vi "Teleop.vi"(10 "Match Info":T2={"Autonomous Elapsed Seconds"=0.0, "TeleOp Elapsed Seconds"=0.0, "Disabled Elapsed Seconds"=0.0, "Visited Autonomous"=FALSE, "Visited TeleOp"=FALSE, "Visited Disabled"=FALSE, "Autonomous Settings"={"Autonomous Style"=enum."Independent", "VI Refnum"=refnum}}, 11 "Call Context":T3) -> ()   [LabVIEW 2016]
doc: "This VI is called for each TeleOp packet received from the DS where the robot is not disabled. It is often used to read from the joysticks and update I/O or to update setpoints for timed control loops. It should complete and return within 20 milliseconds or it may miss DS packets."
uses:
  <vilib>/Rock Robotics/WPI/DriverStation/WPI_DriverStationDerivedRobotMode.ctl
  <vilib>/Rock Robotics/WPI/DriverStation/WPI_DriverStationMatch Info.ctl
  Robot Global Data.vi
  <vilib>/Rock Robotics/WPI/Utilities/WPI_GetSetVariantRefNum.vi
  <vilib>/Rock Robotics/WPI/Solenoid/Deprecated/WPI_SolenoidSetBool.vi
  <vilib>/addons/control/pid/pid.llb/PID (DBL).vi
  navX Library v2/navX Library v2.lvlib
  <vilib>/addons/control/pid/NI_PID_pid.lvlib
panel:
  in  "MOE":dbl=25.0 format="%#_13g"
  in  "Center":dbl=180.0 format="%#_13g"
  out "out left":dbl
  out "out right":dbl
  in  "Pid Factor":dbl=8400.0
  in  "Mode":bool=TRUE
  in  "output range":cluster{"output high":dbl, "output low":dbl}={"output high"=1.0, "output low"=-1.0} {"output low" format="%.2f"; "output high" format="%.2f"}
  in  "PID gains":T1={"proportional gain (Kc)"=0.00021, "integral time (Ti, min)"=15.0, "derivative time (Td, min)"=0.0} {"derivative time (Td, min)" format="%.6f"; "integral time (Ti, min)" format="%.6f"; "proportional gain (Kc)" format="%.6f"}
  out "Left":dbl(graph)
  out "Right":dbl(graph)
  out "Encoder Right":dbl(graph)
  out "Encoder Left":dbl(graph)
  in  "Speed":dbl=0.45 format="%#_13g"
  out "Out Left":dbl(graph)
  out "Out Right":dbl(graph)
  out "Shooter":cluster{"Sensor Velocity":dbl, dbl, dbl}(graph)
  in  "ShooterRPM":dbl
  in  "P":dbl=0.5 format="%#_13g"
  in  "I":dbl format="%#_13g"
  in  "D":dbl format="%#_13g"
  in  "F":dbl=0.005212 format="%#_13g"
  in  "I Zone":dbl format="%#_13g"
  in  "Ramp Rate":dbl format="%#_13g"
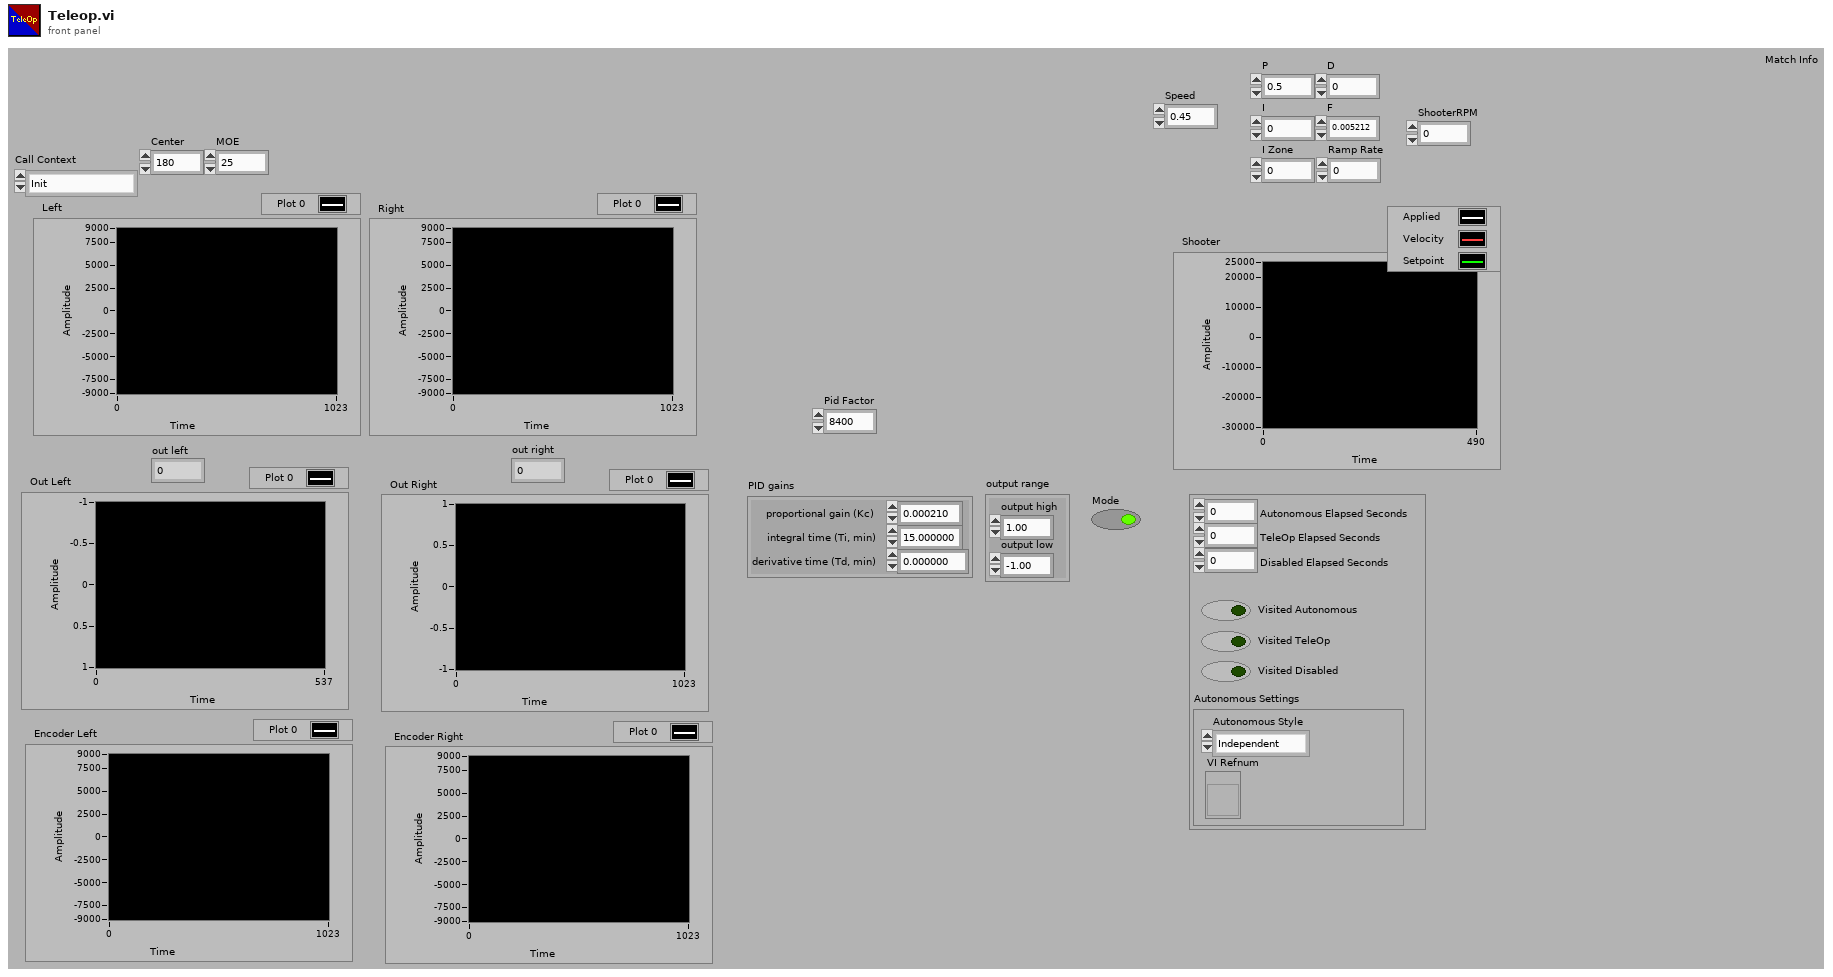
[diagram p1: front panel]
types:
  T1 = cluster{"proportional gain (Kc)":dbl, "integral time (Ti, min)":dbl, "derivative time (Td, min)":dbl}
  T2 = typedef "WPI_DriverStationMatch Info.ctl" = cluster{"Autonomous Elapsed Seconds":dbl, "TeleOp Elapsed Seconds":dbl, "Disabled Elapsed Seconds":dbl, "Visited Autonomous":bool, "Visited TeleOp":bool, "Visited Disabled":bool, "Autonomous Settings":cluster{"Autonomous Style":enum16{"Iterative", "Independent"}, "VI Refnum":refnum<vi>}}
  T3 = typedef "WPI_DriverStationDerivedRobotMode.ctl" = enum16{"Init", "Execute", "Stop"}
  T4 = typedef "WPI_SolenoidDevRef.ctl" = cluster{"DevStatus":errorcluster, "Pneumatics Control Module":u8, "Forward Solenoid Channel":T5, "Reverse Solenoid Channel":T5}
  T5 = typedef "WPI_SolenoidChannel.ctl" = enum8{"Solenoid 0", "Solenoid 1", "Solenoid 2", "Solenoid 3", "Solenoid 4", "Solenoid 5", "Solenoid 6", "Solenoid 7", "Invalid"}
  T6 = typedef "WPI_JoystickDevRef.ctl" = cluster{"Device":T7}
  T7 = typedef "WPI_JoystickDeviceEnum.ctl" = enum16{"USB 0", "USB 1", "USB 2", "USB 3", "USB 4", "USB 5"}
  T8 = cluster{"Buttons[0]":bool, "Buttons[1]":bool, "Buttons[2]":bool, "Buttons[3]":bool, "Buttons[4]":bool, "Buttons[5]":bool, "Buttons[6]":bool, "Buttons[7]":bool, "Buttons[8]":bool}
  T9 = cluster{"Axes[0]":dbl, "Axes[1]":dbl, "Axes[2]":dbl, "Axes[3]":dbl, "Axes[4]":dbl, "Axes[5]":dbl, "Axes[6]":dbl, "Axes[7]":dbl, "Axes[8]":dbl}
  T10 = typedef "navX Library v2.lvlib/Z900_navX_DeviceTypeDef.ctl" = cluster{"Interface":cluster{"Protocol":T11, "Update Rate (4Hz-100Hz)":u8, "navX Open TypeDef":variant}, "Notify Packet":refnum<notifier>, "Loop VI Refnum":refnum<vi>, "Ready to Close Occurrence Refnum":refnum<k4>}
  T11 = typedef "navX Library v2.lvlib/Z900_navX_ProtocolTypeDef.ctl" = enum16{"SERIAL", "I2C", "SPI"}
  T12 = cluster{"Velocity X":dbl, "Velocity Y":dbl, "Velocity Z":dbl, "Displacement X":dbl, "Displacement Y":dbl, "Displacement Z":dbl}
  T13 = cluster{"LinearAcceleration X":dbl, "LinearAcceleration Y":dbl, "LinearAcceleration Z":dbl}
  T14 = cluster{"Yaw":dbl, "Roll":dbl, "Pitch":dbl, "Heading":dbl, "Fused Heading":dbl}
  T15 = typedef "WPI_MotorControlDeviceRef.ctl" = cluster{"DeviceStatus":errorcluster, "Type":T16, "PWM":cluster{"PWM Channel":T17, "DeadBand":T18}, "CAN":cluster{"Device Number":u8, "SetOutput VI Ref":variant, "GetOutput VI Ref":variant, "Enable VI Ref":variant, "Disable VI Ref":variant, "Data":variant}, "Invert":bool}
  T16 = typedef "WPI_MotorControlType.ctl" = enum16{"PWM", "CAN"}
  T17 = typedef "FPGA_DIOPWMChannel.ctl" = enum8{"PWM 0", "PWM 1", "PWM 2", "PWM 3", "PWM 4", "PWM 5", "PWM 6", "PWM 7", "PWM 8", "PWM 9", "PWM MXP 0", "PWM MXP 1", "PWM MXP 2", "PWM MXP 3", "PWM MXP 4", "PWM MXP 5", "PWM MXP 6", "PWM MXP 7", "PWM MXP 8", "PWM MXP 9", "Invalid"}
  T18 = typedef "WPI_PWMDeadband.ctl" = cluster{"Name":string, "maxPositivePwm":i32, "minPositivePwm":i32, "centerPwm":i32, "maxNegativePwm":i32, "minNegativePwm":i32, "angularRange":u16}
  T19 = typedef "WPI_CANTalonSRX_GlobalStatus.ctl" = cluster{"Applied Throttle":dbl, "Module Enabled":bool, "CAN Error":errorcluster, "Closed Loop Error":dbl, "Forward Limit Switch Closed":bool, "Reverse Limit Switch Closed":bool, "Sensor Position":dbl, "Sensor Velocity":dbl, "Current":dbl, "Sticky Fault - Over Temp":bool, "Sticky Fault - Under Voltage":bool, "Sticky Fault - Forward Limit":bool, "Sticky Fault - Reverse Limit":bool, "Sticky Fault - Forward Soft Limit":bool, "Sticky Fault - Reverse Soft Limit":bool, "Brake is Enabled":bool, "Encoder Position":dbl, "Encoder Velocity":dbl, "Encoder Index Count":dbl, "Encoder A Pin State":bool, "Encoder B Pin State":bool, "Encoder Index Pin State":bool, "Analog In":dbl, "Analog In Velocity":dbl, "Temperature (C)":dbl, "Battery Voltage":dbl, "Control 5 Is Supported":bool, "Current Profile Slot Select":dbl, "Pos Div 8":bool, "Vel Div 4":bool, "Pulse Width Position":i32, "Pulse Width Velocity":i32, "Pulse Width Rise To Rise (us)":i32, "Pulse Width Rise To Fall (us)":i32, "Mot Prof Active Is Under Run":bool, "Mot Prof Active Has Under Run":bool, "Mot Prof Active Is Last":bool, "Mot Prof Active Velocity Only":bool, "Mot Prof Active Is Valid":bool, "Mot Prof Buffer Is Full":bool, "Mot Prof Active Profile Slot Select":i32, "Mot Prof NextID":i32, "Mot Prof Count":i32, "Mot Prof Active Velocity":dbl, "Mot Prof Active Position":dbl, "Mot Prof Output Enable":i32}
  T20 = cluster{dbl, "Sensor Velocity":dbl, "ShooterRPM":dbl}
  T21 = typedef "WPI_EncoderDevRef.ctl" = cluster{"DevStatus":errorcluster, "EncoderIndex":T22, "CounterIndex":T23, "DistancePerCount":dbl, "Decoding Type":T24}
  T22 = typedef "FPGA_EncoderIdx.ctl" = enum8{"Enc 0", "Enc 1", "Enc 2", "Enc 3", "Enc 4", "Enc 5", "Enc 6", "Enc 7", "Invalid"}
  T23 = typedef "FPGA_CounterCtrSystemIndex.ctl" = enum8{"Ctr 0", "Ctr 1", "Ctr 2", "Ctr 3", "Ctr 4", "Ctr 5", "Ctr 6", "Ctr 7", "Invalid"}
  T24 = typedef "WPI_EncoderType.ctl" = enum16{"1x", "2x", "4x"}
  T25 = typedef "WPI_RobotDriveDevRef.ctl" = cluster{"DevStatus":errorcluster, "Motors[]":T15[], "Square Inputs":bool, "Max Output":dbl}
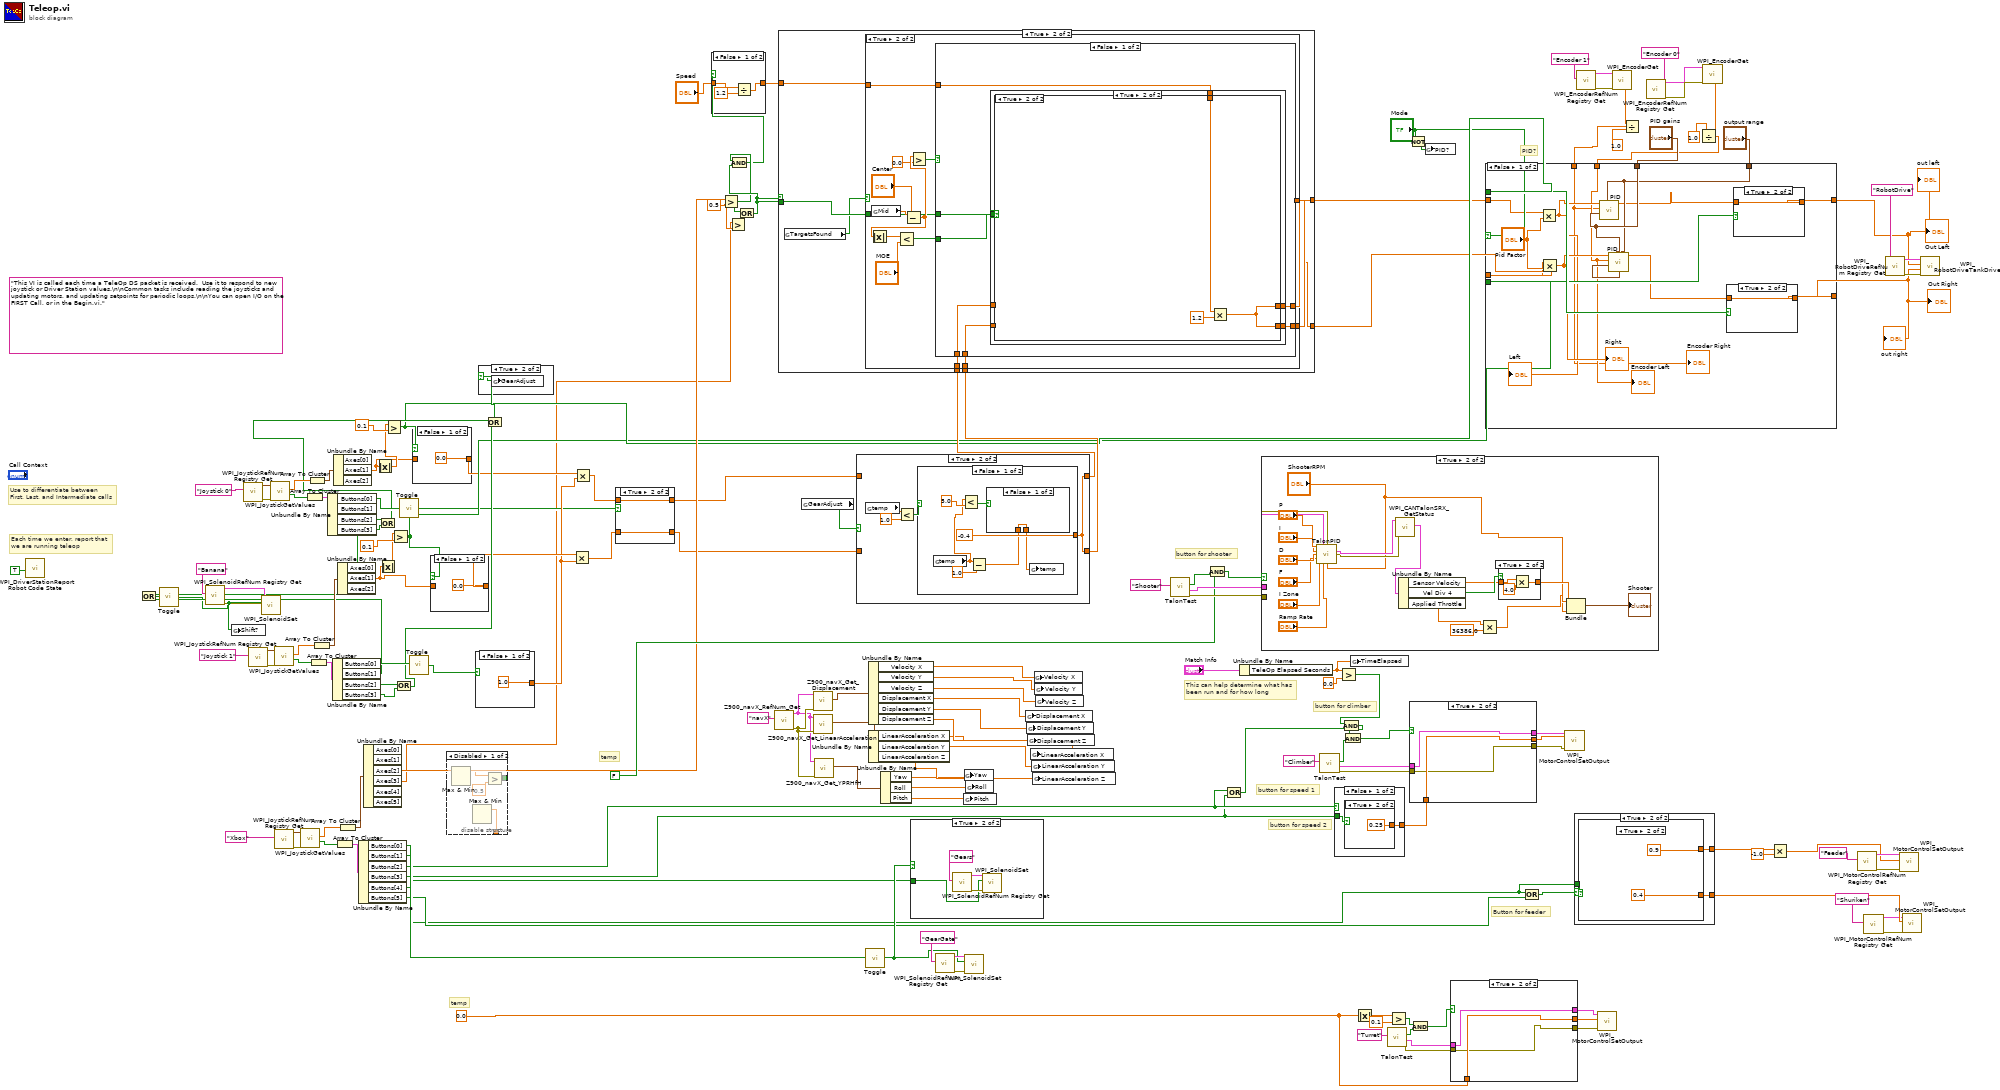
[diagram p0: block diagram]
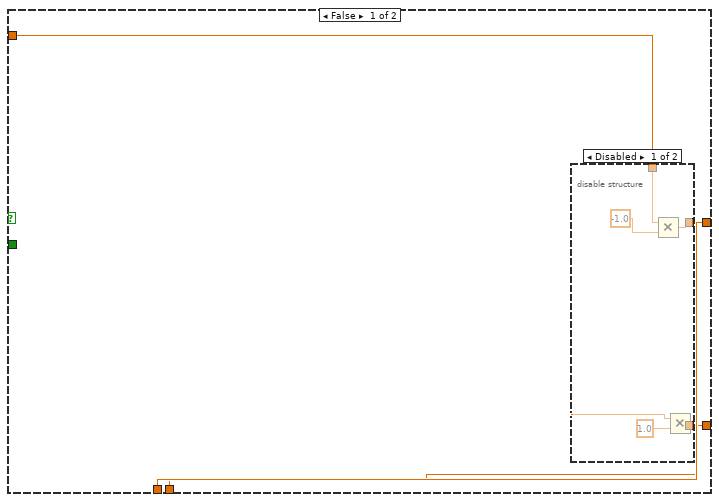
[diagram p4: hidden frame]
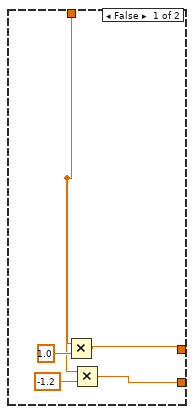
[diagram p7: hidden frame]
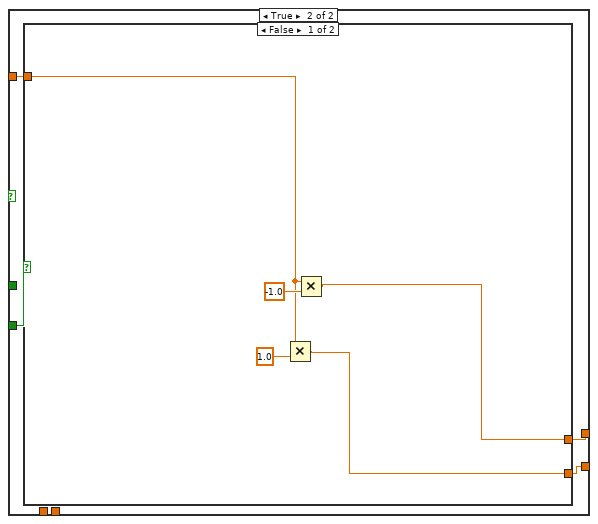
[diagram p8: hidden frame]
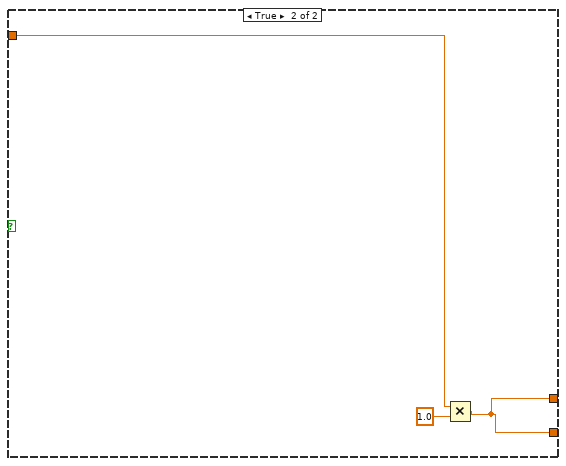
[diagram p9: hidden frame]
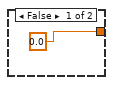
[diagram p10: hidden frame]
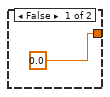
[diagram p11: hidden frame]
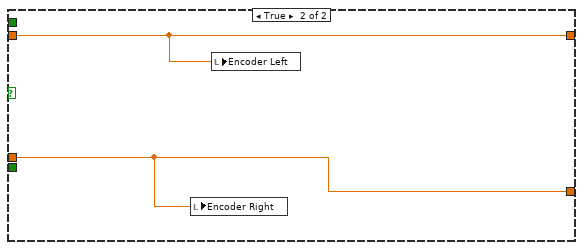
[diagram p12: hidden frame]
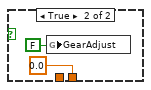
[diagram p16: hidden frame]
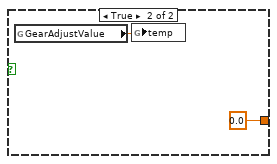
[diagram p17: hidden frame]
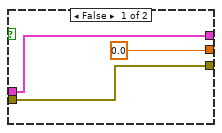
[diagram p18: hidden frame]
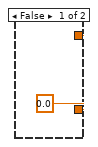
[diagram p20: hidden frame]
diagram:
  w12 = 0.5 ("y")
  w66 = 0.0
  (unwired) "This VI is called each time a TeleOp DS packet is received.  Use it to respond to new joystick or Driver Station values.\n\nCommon tasks include reading the joysticks and updating motors, and updating setpoints for periodic loops.\n\nYou can open I/O on the FIRST Call, or in the Begin.vi."
  # "PID?"
  # "temp"
  # "temp"
  # "Button for feeder"
  # "button for speed 2"
  # "button for speed 1"
  # "button for climber"
  # "button for shooter"
  # "Each time we enter, report that\nwe are running teleop"
  # "Use to differentiate between\nFirst, Last, and Intermediate calls"
  # "This can help determine what has\nbeen run and for how long"
  n1 = call <vilib>:"WPI_DriverStationReport Robot Code State.vi"("TeleOp"=TRUE ("Autonomous")) -> ()  [unwired: 10 in, 1 out]
  n2 = call <vilib>:"WPI_SolenoidRefNum Registry Get.vi"("refnum name"="Banana") -> ("error out"=w20:errorcluster, "SolenoidDevRef"=w19:T4)  [unwired: 9 in]
  n3 = call <vilib>:"WPI_JoystickRefNum Registry Get.vi"("refnum name"="Joystick 0") -> ("error out"=w161:errorcluster, "JoystickDevRef"=w160:T6)  [unwired: 9 in]
  n4 = call <vilib>:"WPI_JoystickRefNum Registry Get.vi"("refnum name"="Joystick 1") -> ("error out"=w153:errorcluster, "JoystickDevRef"=w152:T6)  [unwired: 9 in]
  n5 = call <vilib>:"WPI_JoystickGetValues.vi"("error in (no error)"=w161, "JoystickDevRef"=w160) -> ("Buttons"=w157:bool[], "Axes"=w158:dbl[])  [unwired: 5 in, 3 out]
  n6 = call <vilib>:"WPI_JoystickRefNum Registry Get.vi"("refnum name"="Xbox") -> ("error out"=w113:errorcluster, "JoystickDevRef"=w112:T6)  [unwired: 9 in]
  n7 = call <vilib>:"WPI_JoystickGetValues.vi"("error in (no error)"=w153, "JoystickDevRef"=w152) -> ("Buttons"=w149:bool[], "Axes"=w150:dbl[])  [unwired: 5 in, 3 out]
  n8 = call <vilib>:"WPI_JoystickGetValues.vi"("error in (no error)"=w113, "JoystickDevRef"=w112) -> ("Buttons"=w109:bool[], "Axes"=w110:dbl[])  [unwired: 5 in, 3 out]
  n9 = Array To Cluster(array=w157) -> (cluster=w155:T8)
  n10 = Array To Cluster(array=w158) -> (cluster=w156:T9)
  n11 = Array To Cluster(array=w149) -> (cluster=w147:T8)
  n12 = Array To Cluster(array=w150) -> (cluster=w148:T9)
  n13 = Unbundle By Name(w155) -> ("Buttons[0]"=w141:bool, "Buttons[1]"=w15:bool, "Buttons[2]"=w72:bool, "Buttons[3]"=w71:bool)
  n14 = Unbundle By Name(w147) -> ("Buttons[0]"=w140:bool, "Buttons[1]"=w16:bool, "Buttons[2]"=w74:bool, "Buttons[3]"=w73:bool)
  n15 = Or(x=w15, y=w16) -> (x .or. y?=w17:bool)
  n16 = call "Toggle.vi"("Input"=w17) -> ("Output"=w2:bool)
  n17 = global write "Robot Global Data.vi" "Shift?"(w2) -> ()
  n18 = call-poly <vilib>:"WPI_SolenoidSet.vi"("error in (no error)"=w20, "Value"=w2, "SolenoidDevRef"=w19) -> ()  [unwired: 7 in, 2 out]
  n19 = Unbundle By Name(w156) -> ("Axes[1]"=w142:dbl)  [unwired: 2 out]
  n20 = Array To Cluster(array=w109) -> (cluster=w107:T8)
  n21 = Unbundle By Name(w148) -> ("Axes[1]"=w144:dbl)  [unwired: 2 out]
  n22 = Array To Cluster(array=w110) -> (cluster=w108:T9)
  n23 = Unbundle By Name(w107) -> ("Buttons[0]"=w106:bool, "Buttons[1]"=w105:bool, "Buttons[2]"=w104:bool, "Buttons[3]"=w103:bool, "Buttons[4]"=w100:bool, "Buttons[5]"=w101:bool)
  n24 = Unbundle By Name(w108) -> ("Axes[2]"=w64:dbl, "Axes[3]"=w11:dbl)  [unwired: 4 out]
  n25 = Absolute Value(x=w142) -> (abs(x)=w143:dbl)
  n26 = Or(x=w72, y=w71) -> (x .or. y?=w70:bool)
  n27 = Absolute Value(x=w144) -> (abs(x)=w145:dbl)
  n28 = Greater?(x=w143, y=0.1 ("x")) -> (0:w55:bool)
  n29 = Greater?(x=w145, y=0.1 ("x")) -> (0:w54:bool)
  n30 = Or(x=w74, y=w73) -> (x .or. y?=w69:bool)
  n31 = call "Toggle.vi"("Input"=w141) -> ("Output"=w46:bool)
  n32 = call "Toggle.vi"("Input"=w140) -> ("Output"=w139:bool)
  n33 = case shown="False" w55 {
    tunnel: w142 -> [_ w164]
    tunnel: [0.0 w164] -> w51
    frame False {
    }
    frame True {
    }
  }
  n34 = case shown="False" w54 {
    tunnel: w144 -> [_ w166]
    tunnel: [0.0 w166] -> w53
    frame False {
    }
    frame True {
    }
  }
  n35 = disable-structure shown="Disabled" {
    disable-tunnel: [w168 _] -> _
    disable-tunnel: [w167 _] -> _
    frame Disabled {
      n36 = Max & Min() -> (max(x,y)=w170:dbl)  [unwired: 2 in, 1 out]
      n37 = Max & Min() -> (max(x,y)=w167:dbl)  [unwired: 2 in, 1 out]
      n38 = Greater?(x=w170, y=0.5) -> (0:w168:bool)
    }
    frame Enabled {
    }
  }
  n39 = case shown="False" w139 {
    tunnel: [1.0 0.8] -> w52
    frame False {
    }
    frame True {
    }
  }
  n40 = Or(x=w70, y=w69) -> (x .or. y?=w67:bool)
  n41 = case shown="True" w67 {
    selector: w67 -> [_ w173]
    frame False {
    }
    frame True {
      n42 = global write "Robot Global Data.vi" "GearAdjust"(w173) -> ()
    }
  }
  n43 = Multiply(x=w53, y=w52) -> (x*y=w49:dbl)
  n44 = Multiply(x=w51, y=w52) -> (x*y=w50:dbl)
  n45 = case shown="True" w46 {
    tunnel: w50 -> [w175 w180]
    tunnel: w49 -> [w174 w179]
    tunnel: [w178 w180] -> w48
    tunnel: [w177 w179] -> w47
    frame False {
      w176 = -1.0
      n46 = Multiply(x=w176, y=w175) -> (x*y=w177:dbl)
      n47 = Multiply(x=w174, y=w176) -> (x*y=w178:dbl)
    }
    frame True {
    }
  }
  n48 = Greater?(x=w64, y=w12) -> (0:w6:bool)
  n49 = Greater?(x=w11, y=w12) -> (0:w8:bool)
  n50 = Or(x=w6, y=w8) -> (x .or. y?=w7:bool)
  n51 = And(x=w6, y=w7) -> (x .and. y?=w5:bool)
  n52 = case shown="False" w5 {
    tunnel: [w183 w184] -> w10
    tunnel: "Speed" -> [w182 w184]
    frame False {
      n53 = Divide(x=w182, y=1.2) -> (x/y=w183:dbl)
    }
    frame True {
    }
  }
  n54 = call "Z900_navX_RefNum_Get.vi"("refnum name"="navX") -> ("error out"=w137:errorcluster, "navX Device"=w136:T10)  [unwired: 9 in]
  n55 = global read "Robot Global Data.vi" "GearAdjust"() -> (w68:bool)
  n56 = call "Z900_navX_Get_Displacement.vi"("error in (no error)"=w137, "navX Device"=w136) -> ("Displacement"=w133:T12)  [unwired: 6 in, 3 out]
  n57 = call "Z900_navX_Get_LinearAcceleration.vi"("error in (no error)"=w137, "navX Device"=w136) -> ("Linear Acceleration"=w134:T13)  [unwired: 6 in, 3 out]
  n58 = call "Z900_navX_Get_YPRHfH.vi"("error in (no error)"=w137, "navX Device"=w136) -> ("YRPHfH"=w135:T14)  [unwired: 6 in, 3 out]
  n59 = case shown="True" w68 {
    tunnel: w48 -> [w186 _]
    tunnel: w47 -> [w185 _]
    tunnel: [w186 w187] -> w60
    tunnel: [w185 w187] -> w59
    frame False {
    }
    frame True {
      n60 = global read "Robot Global Data.vi" "temp"() -> (w190:dbl)
      n61 = Less?(x=w190, y=1.0) -> (x < y?=w188:bool)
      n62 = case shown="False" w188 {
        tunnel: [-0.4 0.0] -> w187
        frame False {
          n63 = global read "Robot Global Data.vi" "temp"() -> (w193:dbl)
          n64 = Less?(x=w193, y=5.0 ("x")) -> (x < y?=w194:bool)
          n65 = Subtract(x=w193, y=1.0) -> (x-y=w191:dbl)
          n66 = case shown="False" w194 {
            tunnel: [w198 0.0] -> w192
            tunnel: w191 -> [w198 _]
            frame False {
            }
            frame True {
              n67 = global write "Robot Global Data.vi" "GearAdjust"(FALSE) -> ()
            }
          }
          n68 = global write "Robot Global Data.vi" "temp"(w192) -> ()
        }
        frame True {
          n69 = global read "Robot Global Data.vi" "GearAdjustValue"() -> (w202:dbl)
          n70 = global write "Robot Global Data.vi" "temp"(w202) -> ()
        }
      }
    }
  }
  n71 = case shown="True" w7 {
    tunnel: w60 -> [w204 w211]
    tunnel: w59 -> [w203 w210]
    tunnel: w7 -> [_ w209]
    tunnel: [w204 w207] -> w13
    tunnel: [w203 w206] -> w14
    tunnel: w10 -> [_ w205]
    frame False {
    }
    frame True {
      n72 = global read "Robot Global Data.vi" "TargetsFound"() -> (w208:bool)
      n73 = case shown="True" w208 {
        tunnel: w211 -> [w213 w228]
        tunnel: w210 -> [w212 w227]
        tunnel: [w212 w226] -> w207
        tunnel: [w213 w225] -> w206
        tunnel: w209 -> [_ w221]
        tunnel: w205 -> [w214 w220]
        frame False {
          n74 = disable-structure shown="Disabled" {
            disable-tunnel: [w218 _] -> _
            disable-tunnel: [w217 _] -> _
            disable-tunnel: w214 -> [w215 _]
            frame Disabled {
              n75 = Multiply(x=w215, y=-1.0) -> (x*y=w218:dbl)
              n76 = Multiply(x=w215, y=1.0) -> (x*y=w217:dbl)
            }
            frame Enabled {
            }
          }
        }
        frame True {
          n77 = global read "Robot Global Data.vi" "Mid"() -> (w233:dbl)
          n78 = Subtract(x=w233, y="Center") -> (x-y=w223:dbl)
          n79 = Absolute Value(x=w223) -> (abs(x)=w231:dbl)
          n80 = Less?(x=w231, y="MOE") -> (x < y?=w229:bool)
          n81 = Greater?(x=w223, y=0.0) -> (0:w224:bool)
          n82 = case shown="False" w224 {
            tunnel: w229 -> [w240 w258]
            tunnel: w228 -> [w239 _]
            tunnel: w227 -> [w238 _]
            tunnel: [w237 w256] -> w226
            tunnel: [w236 w257] -> w225
            tunnel: w221 -> [w235 _]
            tunnel: w220 -> [w234 w255]
            frame False {
              n83 = case shown="True" w235 {
                tunnel: w240 -> [_ w246]
                tunnel: w239 -> [w242 _]
                tunnel: w238 -> [w241 _]
                tunnel: [w242 w245] -> w236
                tunnel: [w241 w244] -> w237
                tunnel: w234 -> [_ w243]
                frame False {
                }
                frame True {
                  n84 = case shown="True" w246 {
                    tunnel: [w251 w254] -> w245
                    tunnel: [w249 w254] -> w244
                    tunnel: w243 -> [w247 w252]
                    frame False {
                      n85 = Multiply(x=w247, y=1.0) -> (x*y=w251:dbl)
                      n86 = Multiply(x=w247, y=-1.2) -> (x*y=w249:dbl)
                    }
                    frame True {
                      n87 = Multiply(x=w252, y=1.2) -> (x*y=w254:dbl)
                    }
                  }
                }
              }
            }
            frame True {
              n88 = case shown="False" w258 {
                tunnel: [w263 w266] -> w257
                tunnel: [w261 w266] -> w256
                tunnel: w255 -> [w259 w264]
                frame False {
                  n89 = Multiply(x=w259, y=1.0) -> (x*y=w261:dbl)
                  n90 = Multiply(x=w259, y=-1.0) -> (x*y=w263:dbl)
                }
                frame True {
                  n91 = Multiply(x=w264, y=1.0) -> (x*y=w266:dbl)
                }
              }
            }
          }
        }
      }
    }
  }
  n92 = call "Toggle.vi"("Input"=w106) -> ("Output"=w114:bool)
  n93 = Unbundle By Name(w133) -> ("Velocity X"=w45:dbl, "Velocity Y"=w44:dbl, "Velocity Z"=w43:dbl, "Displacement X"=w42:dbl, "Displacement Y"=w41:dbl, "Displacement Z"=w40:dbl)
  n94 = Unbundle By Name(w134) -> ("LinearAcceleration X"=w39:dbl, "LinearAcceleration Y"=w38:dbl, "LinearAcceleration Z"=w37:dbl)
  n95 = Unbundle By Name(w135) -> ("Yaw"=w36:dbl, "Roll"=w35:dbl, "Pitch"=w34:dbl)
  n96 = case shown="True" w114 {
    tunnel: w105 -> [_ w267]
    frame False {
    }
    frame True {
      n97 = call <vilib>:"WPI_SolenoidRefNum Registry Get.vi"("refnum name"="Gears") -> ("error out"=w270:errorcluster, "SolenoidDevRef"=w269:T4)  [unwired: 9 in]
      n98 = call-poly <vilib>:"WPI_SolenoidSet.vi"("error in (no error)"=w270, "Value"=w267, "SolenoidDevRef"=w269) -> ()  [unwired: 7 in, 2 out]
    }
  }
  n99 = call <vilib>:"WPI_SolenoidRefNum Registry Get.vi"("refnum name"="GearGate") -> ("error out"=w117:errorcluster, "SolenoidDevRef"=w116:T4)  [unwired: 9 in]
  n100 = global write "Robot Global Data.vi" "Pitch"(w34) -> ()
  n101 = global write "Robot Global Data.vi" "Yaw"(w36) -> ()
  n102 = call-poly <vilib>:"WPI_SolenoidSet.vi"("error in (no error)"=w117, "Value"=w114, "SolenoidDevRef"=w116) -> ()  [unwired: 7 in, 2 out]
  n103 = global write "Robot Global Data.vi" "Roll"(w35) -> ()
  n104 = global write "Robot Global Data.vi" "Displacement X"(w42) -> ()
  n105 = global write "Robot Global Data.vi" "Displacement Y"(w41) -> ()
  n106 = global write "Robot Global Data.vi" "Displacement Z"(w40) -> ()
  n107 = global write "Robot Global Data.vi" "LinearAcceleration X"(w39) -> ()
  n108 = global write "Robot Global Data.vi" "LinearAcceleration Y"(w38) -> ()
  n109 = global write "Robot Global Data.vi" "LinearAcceleration Z"(w37) -> ()
  n110 = global write "Robot Global Data.vi" "Velocity X"(w45) -> ()
  n111 = global write "Robot Global Data.vi" "Velocity Y"(w44) -> ()
  n112 = global write "Robot Global Data.vi" "Velocity Z"(w43) -> ()
  n113 = call "TalonTest.vi"("Name"="Shooter") -> ("Output"=w127:bool, "Ref"=w131:T15, "error out"=w130:errorcluster)  [unwired: 7 in]
  n114 = And(x=FALSE, y=w127) -> (x .and. y?=w128:bool)
  n115 = Or(x=w104, y=w103) -> (x .or. y?=w102:bool)
  n116 = Unbundle By Name("Match Info") -> ("TeleOp Elapsed Seconds"=w4:dbl)
  n117 = case shown="True" w128 {
    tunnel: w131 -> [_ w275]
    tunnel: w130 -> [_ w271]
    frame False {
    }
    frame True {
      n118 = call "TalonPID.vi"("P"="P", "Ref In"=w275, "Error in"=w271, "I"="I", "D"="D", "F"="F", "I Zone"="I Zone", "Ramp Rate"="Ramp Rate", "Output"="ShooterRPM") -> ("Ref Out"=w274:T15, "error out"=w273:errorcluster)  [unwired: 5 in]
      n119 = call <vilib>:"WPI_CANTalonSRX_GetStatus.vi"("error in (no error)"=w273, "CAN Talon SRX Ref"=w274) -> ("Talon SRX Status"=w289:T19)  [unwired: 7 in, 2 out]
      n120 = Unbundle By Name(w289) -> ("Sensor Velocity"=w287:dbl, "Vel Div 4"=w288:bool, "Applied Throttle"=w284:dbl)
      n121 = Multiply(x=w284, y=36386.0) -> (x*y=w283:dbl)
      n122 = case shown="True" w288 {
        tunnel: w287 -> [w290 w292]
        tunnel: [w290 w293] -> w282
        frame False {
        }
        frame True {
          n123 = Multiply(x=w292, y=4.0) -> (x*y=w293:dbl)
        }
      }
      n124 = Bundle(w283, "Sensor Velocity"=w282, "ShooterRPM"="ShooterRPM") -> (→"Shooter":T20)  [unwired: 1 in]
    }
  }
  n125 = call "TalonTest.vi"("Name"="Climber") -> ("Output"=w125:bool, "Ref"=w120:T15, "error out"=w119:errorcluster)  [unwired: 7 in]
  n126 = case shown="False" w104 {
    tunnel: [w295 w299] -> w118
    tunnel: w103 -> [w294 w298]
    frame False {
      n127 = case shown="True" w294 {
        tunnel: [0.0 0.25] -> w295
        frame False {
        }
        frame True {
        }
      }
    }
    frame True {
      n128 = case shown="True" w298 {
        tunnel: [0.75 1.0] -> w299
        frame False {
        }
        frame True {
        }
      }
    }
  }
  n129 = Greater?(x=w4, y=0.0) -> (0:w122:bool)
  n130 = And(x=w122, y=w102) -> (x .and. y?=w126:bool)
  n131 = And(x=w126, y=w125) -> (x .and. y?=w121:bool)
  n132 = global write "Robot Global Data.vi" "TimeElapsed"(w4) -> ()
  n133 = Absolute Value(x=w66) -> (abs(x)=w93:dbl)
  n134 = call "TalonTest.vi"("Name"="Turret") -> ("Output"=w97:bool, "Ref"=w95:T15, "error out"=w94:errorcluster)  [unwired: 7 in]
  n135 = Greater?(x=w93, y=0.1) -> (0:w91:bool)
  n136 = Not(x="Mode") -> (.not. x?=w1:bool)
  n137 = case shown="True" w121 {
    tunnel: w120 -> [w303 w307]
    tunnel: w119 -> [w302 w305]
    tunnel: w118 -> [_ w306]
    tunnel: [w303 w307] -> w86
    tunnel: [0.0 w306] -> w87
    tunnel: [w302 w305] -> w85
    frame False {
    }
    frame True {
    }
  }
  n138 = And(x=w91, y=w97) -> (x .and. y?=w96:bool)
  n139 = global write "Robot Global Data.vi" "PID?"(w1) -> ()
  n140 = case shown="True" w96 {
    tunnel: w95 -> [w309 w313]
    tunnel: w94 -> [w308 w311]
    tunnel: w66 -> [_ w312]
    tunnel: [w309 w313] -> w90
    tunnel: [0.0 w312] -> w89
    tunnel: [w308 w311] -> w88
    frame False {
    }
    frame True {
    }
  }
  n141 = Or(x=w100, y=w101) -> (x .or. y?=w99:bool)
  n142 = call <vilib>:"WPI_MotorControlSetOutput.vi"("error in (no error)"=w85, "Output"=w87, "MotorControlDevRef"=w86) -> ()  [unwired: 6 in, 3 out]
  n143 = case shown="True" w99 {
    tunnel: w100 -> [_ w317]
    tunnel: [w314 w316] -> w77
    tunnel: [w314 w315] -> w84
    frame False {
      w314 = 0.0
    }
    frame True {
      n144 = case shown="True" w317 {
        tunnel: [-0.9 ("Output") 0.9 ("Output")] -> w316
        tunnel: [-0.4 ("Output") 0.4 ("Output")] -> w315
        frame False {
        }
        frame True {
        }
      }
    }
  }
  n145 = call <vilib>:"WPI_EncoderRefNum Registry Get.vi"("refnum name"="Encoder 1") -> ("error out"=w33:errorcluster, "EncoderDevRef"=w32:T21)  [unwired: 9 in]
  n146 = call <vilib>:"WPI_MotorControlSetOutput.vi"("error in (no error)"=w88, "Output"=w89, "MotorControlDevRef"=w90) -> ()  [unwired: 6 in, 3 out]
  n147 = call <vilib>:"WPI_EncoderGet.vi"("error in (no error)"=w33, "EncoderDevRef"=w32) -> ("Rate"=w23:dbl)  [unwired: 4 in, 5 out]
  n148 = Divide(x=w23, y=1.0) -> (x/y=w26:dbl)
  n149 = call <vilib>:"WPI_EncoderRefNum Registry Get.vi"("refnum name"="Encoder 0") -> ("error out"=w30:errorcluster, "EncoderDevRef"=w29:T21)  [unwired: 9 in]
  n150 = call <vilib>:"WPI_EncoderGet.vi"("error in (no error)"=w30, "EncoderDevRef"=w29) -> ("Rate"=w25:dbl)  [unwired: 4 in, 5 out]
  n151 = Divide(x=w25, y=1.0) -> (x/y=w27:dbl)
  n152 = case shown="False" "Mode" {
    tunnel: w13 -> [w327 w342]
    tunnel: w14 -> [w326 w341]
    tunnel: w26 -> [w322 _]
    tunnel: w27 -> [w323 _]
    tunnel: "PID gains" -> [w336 _]
    tunnel: "output range" -> [w335 _]
    tunnel: w55 -> [w332 _]
    tunnel: w54 -> [w331 _]
    tunnel: [w333 w341] -> w57
    tunnel: [w334 w342] -> w21
    frame False {
      n153 = Multiply(x=w327, y="Pid Factor") -> (x*y=w324:dbl)
      "Left" <- w324
      n154 = Multiply(x=w326, y="Pid Factor") -> (x*y=w325:dbl)
      "Right" <- w325
      n155 = call-poly <vilib>:"PID.vi"("output range"=w335, "PID gains"=w336, "process variable"=w322, "setpoint"=w324) -> ("output"=w330:dbl)  [unwired: 6 in, 1 out]
      n156 = call-poly <vilib>:"PID.vi"("output range"=w335, "PID gains"=w336, "process variable"=w323, "setpoint"=w325) -> ("output"=w329:dbl)  [unwired: 6 in, 1 out]
      n157 = case shown="True" w332 {
        tunnel: w329 -> [_ w338]
        tunnel: [0.0 w338] -> w333
        frame False {
        }
        frame True {
        }
      }
      n158 = case shown="True" w331 {
        tunnel: w330 -> [_ w340]
        tunnel: [0.0 w340] -> w334
        frame False {
        }
        frame True {
        }
      }
      "Encoder Right" <- w322
      "Encoder Left" <- w323
    }
    frame True {
      n159 = local write "Encoder Right"(w341) -> ()
      n160 = local write "Encoder Left"(w342) -> ()
    }
  }
  "Out Right" <- w57
  "Out Left" <- w21
  "out right" <- w57
  "out left" <- w21
  n161 = Multiply(x=w77, y=-1.0) -> (x*y=w75:dbl)
  n162 = call <vilib>:"WPI_MotorControlRefNum Registry Get.vi"("refnum name"="Feeder") -> ("error out"=w78:errorcluster, "MotorControlDevRef"=w79:T15)  [unwired: 9 in]
  n163 = call <vilib>:"WPI_MotorControlRefNum Registry Get.vi"("refnum name"="Shuriken") -> ("error out"=w80:errorcluster, "MotorControlDevRef"=w81:T15)  [unwired: 9 in]
  n164 = call <vilib>:"WPI_RobotDriveRefNum Registry Get.vi"("refnum name"="RobotDrive") -> ("error out"=w63:errorcluster, "RobotDriveDevRef"=w62:T25)  [unwired: 9 in]
  n165 = call <vilib>:"WPI_MotorControlSetOutput.vi"("error in (no error)"=w78, "Output"=w75, "MotorControlDevRef"=w79) -> ()  [unwired: 6 in, 3 out]
  n166 = call <vilib>:"WPI_MotorControlSetOutput.vi"("error in (no error)"=w80, "Output"=w84, "MotorControlDevRef"=w81) -> ()  [unwired: 6 in, 3 out]
  n167 = call <vilib>:"WPI_RobotDriveTankDrive.vi"("error in (no error)"=w63, "Right axis value"=w57, "Left axis value"=w21, "RobotDriveDevRef"=w62) -> ()  [unwired: 5 in, 3 out]
